vi "uTTA_SetPGAGain.vi"(5 "Mode":T1, 8 "error in":errorcluster, 10 "PGA Gain":u16 max=3, 11 "VISA Refnum in":refnum<visa-resource-name>) -> (0 "error out":errorcluster, 3 "VISA Refnum out":refnum<visa-resource-name>, 4 "Set PGA Gain":u32, 7 "Received":string)   [LabVIEW 2021]
uses:
  uTTA_Controls/CTL_uTTA_PGA_Gain.ctl
panel:
  out "Heating PGA Gain":u32
  out "Cooling PGA Gain":u32
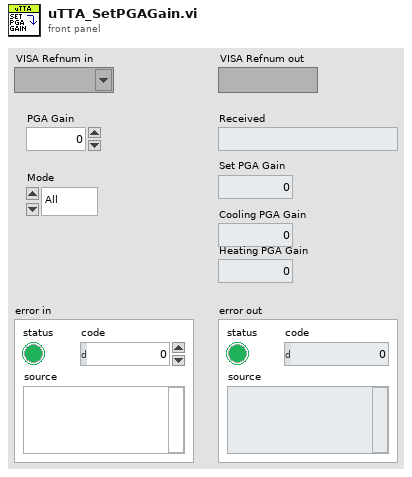
[diagram p1: front panel]
types:
  T1 = typedef "CTL_uTTA_PGA_Gain.ctl" = enum16{"All", "Cooling", "Heating"}
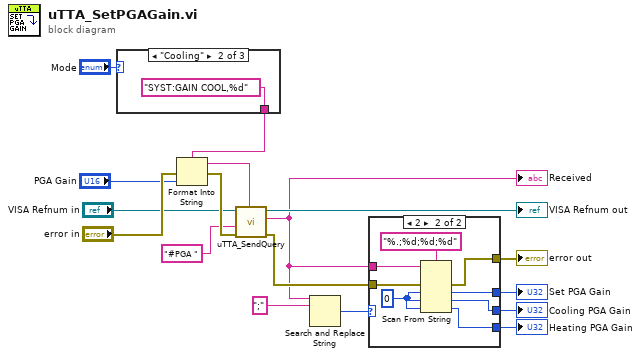
[diagram p0: block diagram]
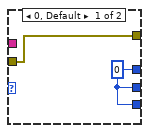
[diagram p2: hidden frame]
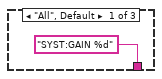
[diagram p3: hidden frame]
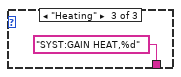
[diagram p4: hidden frame]
diagram:
  n1 = case shown="\"Cooling\"" "Mode" {
    tunnel: ["SYST:GAIN %d" ("format string") "SYST:GAIN COOL,%d" ("format string") "SYST:GAIN HEAT,%d" ("format string")] -> w7
    frame "All", Default {
    }
    frame "Cooling" {
    }
    frame "Heating" {
    }
  }
  n2 = Format Into String(format string=w7, error in="error in", "PGA Gain") -> (resulting string=w13:string, error out=w15:errorcluster)  [unwired: 1 in]
  n3 = call "uTTA_SendQuery.vi"("Send String"=w13, "error in (no error)"=w15, "Response Qualifier(\"\")"="#PGA " ("Response Qualifier(\"\")"), "VISA Refnum in"="VISA Refnum in") -> ("error out"=w16:errorcluster, "Received"=w4:string, "VISA Refnum out"=→"VISA Refnum out":refnum<visa-resource-name>)  [unwired: 5 in]
  "Received" <- w4
  n4 = Search and Replace String(input string=w4, search string=";") -> (number of replacements=w2:i32)  [unwired: 6 in, 3 out]
  n5 = case shown="2" w2 {
    tunnel: [w22 w30] -> w17
    tunnel: w16 -> [w22 w29]
    tunnel: [w21 w27] -> w9
    tunnel: [w21 w25] -> w6
    tunnel: [w21 w24] -> w5
    tunnel: w4 -> [_ w23]
    frame 0, Default {
      w21 = u32 0 ("default value 1")
    }
    frame 2 {
      w26 = u32 0 ("default value 1")
      n6 = Scan From String(format string="%.;%d;%d;%d", input string=w23, error in=w29, default 1=w26, default 2=w26, default 3=w26) -> (error out=w30:errorcluster, output 1=w27:u32, output 2=w25:u32, output 3=w24:u32)  [unwired: 1 in, 2 out]
    }
  }
  "Set PGA Gain" <- w9
  "error out" <- w17
  "Cooling PGA Gain" <- w6
  "Heating PGA Gain" <- w5
